vi "Write named settings.vi"(7 "Names":string[](array[string]), 8 "error in (no error)":errorcluster, 10 "VI ref":refnum<vi>, 11 "refnum":T1) -> (0 "error out":errorcluster, 3 "refnum out":T1)   [LabVIEW 2018]
uses:
  <vilib>/Utility/config.llb/Config Data RefNum.ctl
  <vilib>/Utility/config.llb/NI_LVConfig.lvlib
panel:
  in  "float number format (optional)":string
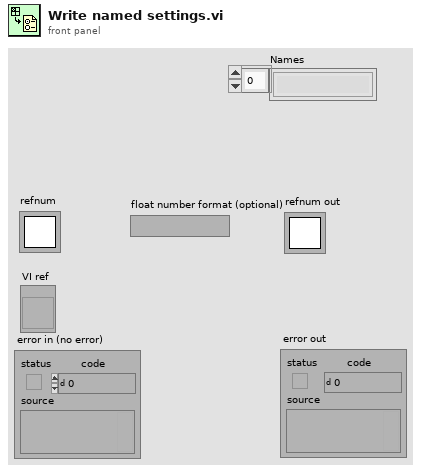
[diagram p1: front panel]
types:
  T1 = typedef "NI_LVConfig.lvlib/Config Data RefNum.ctl" = refnum<k1>
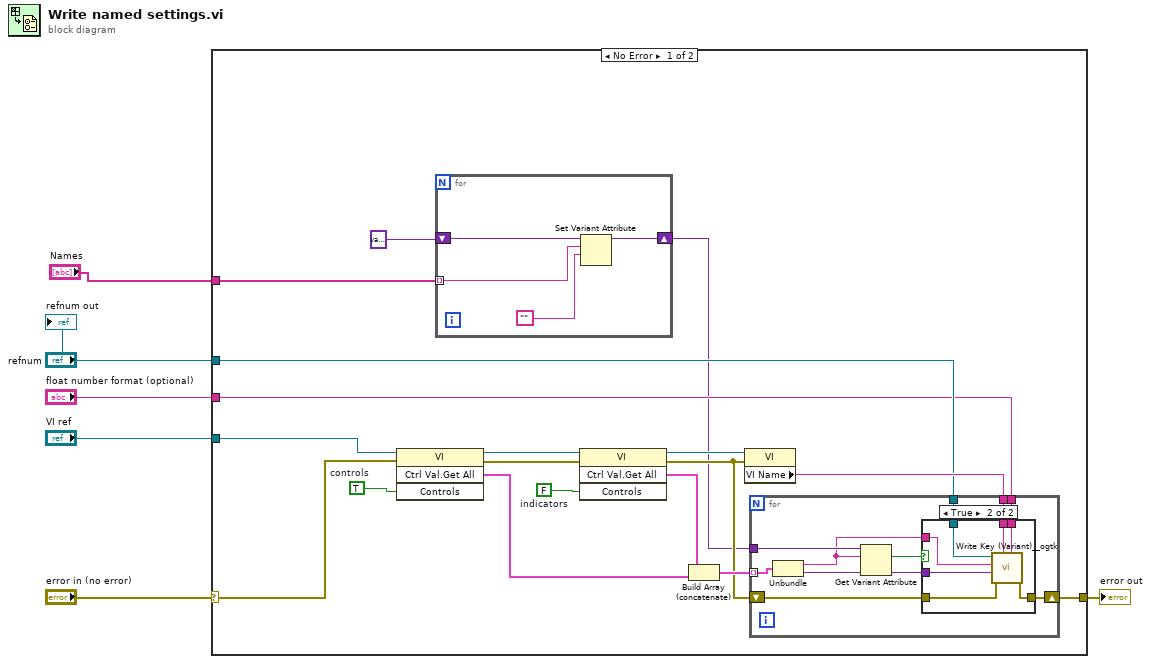
[diagram p0: block diagram]
diagram:
  n1 = case shown="No Error" "error in (no error)" {
    selector: "error in (no error)" -> [w11 w47]
    tunnel: "refnum" -> [w15 _]
    tunnel: [w13 w47] -> w5
    tunnel: "VI ref" -> [w12 _]
    tunnel: "float number format (optional)" -> [w10 _]
    tunnel: "Names" -> [w7 _]
    frame No Error {
      w22 = FALSE  # indicators
      w24 = TRUE  # controls
      n2 = invoke class="VI" method="Ctrl Val.Get All"(reference=w12, error in=w11, "Controls"=w24) -> (reference out=w23:refnum<vi>, error out=w18:errorcluster, "Get All Control Values Variant"=w20:cluster{"Name":string, "Variant Data":variant}[])  [unwired: 1 in, 1 out]
      n3 = for {
        shift-right: [w27] -> w8
        shift-left: variant -> [w28]
        tunnel: w7 -> [w25] mode=indexing
        n4 = Set Variant Attribute(Variant=w28, name=w25, value="") -> (Variant out=w27:variant)  [unwired: 1 in, 2 out]
      }
      n5 = invoke class="VI" method="Ctrl Val.Get All"(reference=w23, error in=w18, "Controls"=w22) -> (reference out=w19:refnum<vi>, error out=w14:errorcluster, "Get All Control Values Variant"=w21:cluster{"Name":string, "Variant Data":variant}[])  [unwired: 1 in, 1 out]
      n6 = Build Array (concatenate)(w21, w20) -> (w17:cluster{"Name":string, "Variant Data":variant}[])
      n7 = property class="VI"(reference=w19, error in=w14) -> ("VI Name"=w16:string)  [unwired: 2 out]
      n8 = for {
        tunnel: w17 -> [w38] mode=indexing
        tunnel: w16 -> [w37]
        tunnel: w15 -> [w36]
        shift-right: [w35] -> w13
        shift-left: w14 -> [w32]
        tunnel: w10 -> [w34]
        tunnel: w8 -> [w30]
        n9 = Unbundle(w38) -> ("Name"=w29:string, "Variant Data"=w33:variant)
        n10 = Get Variant Attribute(Variant=w30, name=w29) -> (found=w31:bool)  [unwired: 2 in, 3 out]
        n11 = case shown="True" w31 {
          tunnel: w37 -> [_ w46]
          tunnel: w36 -> [_ w45]
          tunnel: [w39 w44] -> w35
          tunnel: w34 -> [_ w43]
          tunnel: w33 -> [_ w42]
          tunnel: w32 -> [w39 w41]
          tunnel: w29 -> [_ w40]
          frame False {
          }
          frame True {
            n12 = call <userlib>:"Write Key (Variant)__ogtk.vi"("float number format"=w43, "section"=w46, "error in (no error)"=w41, "key-value"=w42, "key (optional)"=w40, "refnum"=w45) -> ("error out"=w44:errorcluster)  [unwired: 4 in, 1 out]
          }
        }
      }
    }
    frame Error {
    }
  }
  "error out" <- w5
  "refnum out" <- "refnum"
